vi "DevScripts_FlagToRing-Keycode.vi"() -> ()   [LabVIEW 2024]
uses:
  <vilib>/regexp/Match Regular Expression.xnode
panel:
  in  "flags (0)":u32(ring) items=["SDLK_UNKNOWN"=0, "SDLK_RETURN"=13, "SDLK_ESCAPE"=27, "SDLK_BACKSPACE"=8, "SDLK_TAB"=9, "SDLK_SPACE"=32, "SDLK_EXCLAIM"=33, "SDLK_DBLAPOSTROPHE"=34, "SDLK_HASH"=35, "SDLK_DOLLAR"=36, "SDLK_PERCENT"=37, "SDLK_AMPERSAND"=38, "SDLK_APOSTROPHE"=39, "SDLK_LEFTPAREN"=40, "SDLK_RIGHTPAREN"=41, "SDLK_ASTERISK"=42, "SDLK_PLUS"=43, "SDLK_COMMA"=44, "SDLK_MINUS"=45, "SDLK_PERIOD"=46, "SDLK_SLASH"=47, "SDLK_0"=48, "SDLK_1"=49, "SDLK_2"=50, "SDLK_3"=51, "SDLK_4"=52, "SDLK_5"=53, "SDLK_6"=54, "SDLK_7"=55, "SDLK_8"=56, "SDLK_9"=57, "SDLK_COLON"=58, "SDLK_SEMICOLON"=59, "SDLK_LESS"=60, "SDLK_EQUALS"=61, "SDLK_GREATER"=62, "SDLK_QUESTION"=63, "SDLK_AT"=64, "SDLK_LEFTBRACKET"=91, "SDLK_BACKSLASH"=92, "SDLK_RIGHTBRACKET"=93, "SDLK_CARET"=94, "SDLK_UNDERSCORE"=95, "SDLK_GRAVE"=96, "SDLK_A"=97, "SDLK_B"=98, "SDLK_C"=99, "SDLK_D"=100, "SDLK_E"=101, "SDLK_F"=102, "SDLK_G"=103, "SDLK_H"=104, "SDLK_I"=105, "SDLK_J"=106, "SDLK_K"=107, "SDLK_L"=108, "SDLK_M"=109, "SDLK_N"=110, "SDLK_O"=111, "SDLK_P"=112, "SDLK_Q"=113, "SDLK_R"=114, "SDLK_S"=115, "SDLK_T"=116, "SDLK_U"=117, "SDLK_V"=118, "SDLK_W"=119, "SDLK_X"=120, "SDLK_Y"=121, "SDLK_Z"=122, "SDLK_LEFTBRACE"=123, "SDLK_PIPE"=124, "SDLK_RIGHTBRACE"=125, "SDLK_TILDE"=126, "SDLK_DELETE"=127, "SDLK_PLUSMINUS"=177, "SDLK_CAPSLOCK"=1073741881, "SDLK_F1"=1073741882, "SDLK_F2"=1073741883, "SDLK_F3"=1073741884, "SDLK_F4"=1073741885, "SDLK_F5"=1073741886, "SDLK_F6"=1073741887, "SDLK_F7"=1073741888, "SDLK_F8"=1073741889, "SDLK_F9"=1073741890, "SDLK_F10"=1073741891, "SDLK_F11"=1073741892, "SDLK_F12"=1073741893, "SDLK_PRINTSCREEN"=1073741894, "SDLK_SCROLLLOCK"=1073741895, "SDLK_PAUSE"=1073741896, "SDLK_INSERT"=1073741897, "SDLK_HOME"=1073741898, "SDLK_PAGEUP"=1073741899, "SDLK_END"=1073741901, "SDLK_PAGEDOWN"=1073741902, "SDLK_RIGHT"=1073741903, "SDLK_LEFT"=1073741904, "SDLK_DOWN"=1073741905, "SDLK_UP"=1073741906, "SDLK_NUMLOCKCLEAR"=1073741907, "SDLK_KP_DIVIDE"=1073741908, "SDLK_KP_MULTIPLY"=1073741909, "SDLK_KP_MINUS"=1073741910, "SDLK_KP_PLUS"=1073741911, "SDLK_KP_ENTER"=1073741912, "SDLK_KP_1"=1073741913, "SDLK_KP_2"=1073741914, "SDLK_KP_3"=1073741915, "SDLK_KP_4"=1073741916, "SDLK_KP_5"=1073741917, "SDLK_KP_6"=1073741918, "SDLK_KP_7"=1073741919, "SDLK_KP_8"=1073741920, "SDLK_KP_9"=1073741921, "SDLK_KP_0"=1073741922, "SDLK_KP_PERIOD"=1073741923, "SDLK_APPLICATION"=1073741925, "SDLK_POWER"=1073741926, "SDLK_KP_EQUALS"=1073741927, "SDLK_F13"=1073741928, "SDLK_F14"=1073741929, "SDLK_F15"=1073741930, "SDLK_F16"=1073741931, "SDLK_F17"=1073741932, "SDLK_F18"=1073741933, "SDLK_F19"=1073741934, "SDLK_F20"=1073741935, "SDLK_F21"=1073741936, "SDLK_F22"=1073741937, "SDLK_F23"=1073741938, "SDLK_F24"=1073741939, "SDLK_EXECUTE"=1073741940, "SDLK_HELP"=1073741941, "SDLK_MENU"=1073741942, "SDLK_SELECT"=1073741943, "SDLK_STOP"=1073741944, "SDLK_AGAIN"=1073741945, "SDLK_UNDO"=1073741946, "SDLK_CUT"=1073741947, "SDLK_COPY"=1073741948, "SDLK_PASTE"=1073741949, "SDLK_FIND"=1073741950, "SDLK_MUTE"=1073741951, "SDLK_VOLUMEUP"=1073741952, "SDLK_VOLUMEDOWN"=1073741953, "SDLK_KP_COMMA"=1073741957, "SDLK_KP_EQUALSAS400"=1073741958, "SDLK_ALTERASE"=1073741977, "SDLK_SYSREQ"=1073741978, "SDLK_CANCEL"=1073741979, "SDLK_CLEAR"=1073741980, "SDLK_PRIOR"=1073741981, "SDLK_RETURN2"=1073741982, "SDLK_SEPARATOR"=1073741983, "SDLK_OUT"=1073741984, "SDLK_OPER"=1073741985, "SDLK_CLEARAGAIN"=1073741986, "SDLK_CRSEL"=1073741987, "SDLK_EXSEL"=1073741988, "SDLK_KP_00"=1073742000, "SDLK_KP_000"=1073742001, "SDLK_THOUSANDSSEPARATOR"=1073742002, "SDLK_DECIMALSEPARATOR"=1073742003, "SDLK_CURRENCYUNIT"=1073742004, "SDLK_CURRENCYSUBUNIT"=1073742005, "SDLK_KP_LEFTPAREN"=1073742006, "SDLK_KP_RIGHTPAREN"=1073742007, "SDLK_KP_LEFTBRACE"=1073742008, "SDLK_KP_RIGHTBRACE"=1073742009, "SDLK_KP_TAB"=1073742010, "SDLK_KP_BACKSPACE"=1073742011, "SDLK_KP_A"=1073742012, "SDLK_KP_B"=1073742013, "SDLK_KP_C"=1073742014, "SDLK_KP_D"=1073742015, "SDLK_KP_E"=1073742016, "SDLK_KP_F"=1073742017, "SDLK_KP_XOR"=1073742018, "SDLK_KP_POWER"=1073742019, "SDLK_KP_PERCENT"=1073742020, "SDLK_KP_LESS"=1073742021, "SDLK_KP_GREATER"=1073742022, "SDLK_KP_AMPERSAND"=1073742023, "SDLK_KP_DBLAMPERSAND"=1073742024, "SDLK_KP_VERTICALBAR"=1073742025, "SDLK_KP_DBLVERTICALBAR"=1073742026, "SDLK_KP_COLON"=1073742027, "SDLK_KP_HASH"=1073742028, "SDLK_KP_SPACE"=1073742029, "SDLK_KP_AT"=1073742030, "SDLK_KP_EXCLAM"=1073742031, "SDLK_KP_MEMSTORE"=1073742032, "SDLK_KP_MEMRECALL"=1073742033, "SDLK_KP_MEMCLEAR"=1073742034, "SDLK_KP_MEMADD"=1073742035, "SDLK_KP_MEMSUBTRACT"=1073742036, "SDLK_KP_MEMMULTIPLY"=1073742037, "SDLK_KP_MEMDIVIDE"=1073742038, "SDLK_KP_PLUSMINUS"=1073742039, "SDLK_KP_CLEAR"=1073742040, "SDLK_KP_CLEARENTRY"=1073742041, "SDLK_KP_BINARY"=1073742042, "SDLK_KP_OCTAL"=1073742043, "SDLK_KP_DECIMAL"=1073742044, "SDLK_KP_HEXADECIMAL"=1073742045, "SDLK_LCTRL"=1073742048, "SDLK_LSHIFT"=1073742049, "SDLK_LALT"=1073742050, "SDLK_LGUI"=1073742051, "SDLK_RCTRL"=1073742052, "SDLK_RSHIFT"=1073742053, "SDLK_RALT"=1073742054, "SDLK_RGUI"=1073742055, "SDLK_MODE"=1073742081, "SDLK_SLEEP"=1073742082, "SDLK_WAKE"=1073742083, "SDLK_CHANNEL_INCREMENT"=1073742084, "SDLK_CHANNEL_DECREMENT"=1073742085, "SDLK_MEDIA_PLAY"=1073742086, "SDLK_MEDIA_PAUSE"=1073742087, "SDLK_MEDIA_RECORD"=1073742088, "SDLK_MEDIA_FAST_FORWARD"=1073742089, "SDLK_MEDIA_REWIND"=1073742090, "SDLK_MEDIA_NEXT_TRACK"=1073742091, "SDLK_MEDIA_PREVIOUS_TRACK"=1073742092, "SDLK_MEDIA_STOP"=1073742093, "SDLK_MEDIA_EJECT"=1073742094, "SDLK_MEDIA_PLAY_PAUSE"=1073742095, "SDLK_MEDIA_SELECT"=1073742096, "SDLK_AC_NEW"=1073742097, "SDLK_AC_OPEN"=1073742098, "SDLK_AC_CLOSE"=1073742099, "SDLK_AC_EXIT"=1073742100, "SDLK_AC_SAVE"=1073742101, "SDLK_AC_PRINT"=1073742102, "SDLK_AC_PROPERTIES"=1073742103, "SDLK_AC_SEARCH"=1073742104, "SDLK_AC_HOME"=1073742105, "SDLK_AC_BACK"=1073742106, "SDLK_AC_FORWARD"=1073742107, "SDLK_AC_STOP"=1073742108, "SDLK_AC_REFRESH"=1073742109, "SDLK_AC_BOOKMARKS"=1073742110, "SDLK_SOFTLEFT"=1073742111, "SDLK_SOFTRIGHT"=1073742112, "SDLK_CALL"=1073742113, "SDLK_ENDCALL"=1073742114]
  in  "#Define list":string="#define SDLK_SCANCODE_MASK          (1u<<30)\n#define SDL_SCANCODE_TO_KEYCODE(X)  (X | SDLK_SCANCODE_MASK)\n#define SDLK_UNKNOWN                0x00000000u /**< 0 */\n#define SDLK_RETURN                 0x0000000du /**< '\\r' */\n#define SDLK_ESCAPE                 0x0000001bu /**< '\\x1B' */\n#define SDLK_BACKSPACE              0x00000008u /**< '\\b' */\n#define SDLK_TAB                    0x00000009u /**< '\\t' */\n#define SDLK_SPACE                  0x00000020u /**< ' ' */\n#define SDLK_EXCLAIM                0x00000021u /**< '!' */\n#define SDLK_DBLAPOSTROPHE          0x00000022u /**< '\"' */\n#define SDLK_HASH                   0x00000023u /**< '#' */\n#define SDLK_DOLLAR                 0x00000024u /**< '$' */\n#define SDLK_PERCENT                0x00000025u /**< '%' */\n#define SDLK_AMPERSAND              0x00000026u /**< '&' */\n#define SDLK_APOSTROPHE             0x00000027u /**< '\\'' */\n#define SDLK_LEFTPAREN              0x00000028u /**< '(' */\n#define SDLK_RIGHTPAREN             0x00000029u /**< ')' */\n#define SDLK_ASTERISK               0x0000002au /**< '*' */\n#define SDLK_PLUS                   0x0000002bu /**< '+' */\n#define SDLK_COMMA                  0x0000002cu /**< ',' */\n#define SDLK_MINUS                  0x0000002du /**< '-' */\n#define SDLK_PERIOD                 0x0000002eu /**< '.' */\n#define SDLK_SLASH                  0x0000002fu /**< '/' */\n#define SDLK_0                      0x00000030u /**< '0' */\n#define SDLK_1                      0x00000031u /**< '1' */\n#define SDLK_2                      0x00000032u /**< '2' */\n#define SDLK_3                      0x00000033u /**< '3' */\n#define SDLK_4                      0x00000034u /**< '4' */\n#define SDLK_5                      0x00000035u /**< '5' */\n#define SDLK_6                      0x00000036u /**< '6' */\n#define SDLK_7                      0x00000037u /**< '7' */\n#define SDLK_8                      0x00000038u /**< '8' */\n#define SDLK_9                      0x00000039u /**< '9' */\n#define SDLK_COLON                  0x0000003au /**< ':' */\n#define SDLK_SEMICOLON              0x0000003bu /**< ';' */\n#define SDLK_LESS                   0x0000003cu /**< '<' */\n#define SDLK_EQUALS                 0x0000003du /**< '=' */\n#define SDLK_GREATER                0x0000003eu /**< '>' */\n#define SDLK_QUESTION               0x0000003fu /**< '?' */\n#define SDLK_AT                     0x00000040u /**< '@' */\n#define SDLK_LEFTBRACKET            0x0000005bu /**< '[' */\n#define SDLK_BACKSLASH              0x0000005cu /**< '\\\\' */\n#define SDLK_RIGHTBRACKET           0x0000005du /**< ']' */\n#define SDLK_CARET                  0x0000005eu /**< '^' */\n#define SDLK_UNDERSCORE             0x0000005fu /**< '_' */\n#define SDLK_GRAVE                  0x00000060u /**< '`' */\n#define SDLK_A                      0x00000061u /**< 'a' */\n#define SDLK_B                      0x00000062u /**< 'b' */\n#define SDLK_C                      0x00000063u /**< 'c' */\n#define SDLK_D                      0x00000064u /**< 'd' */\n#define SDLK_E                      0x00000065u /**< 'e' */\n#define SDLK_F                      0x00000066u /**< 'f' */\n#define SDLK_G                      0x00000067u /**< 'g' */\n#define SDLK_H                      0x00000068u /**< 'h' */\n#define SDLK_I                      0x00000069u /**< 'i' */\n#define SDLK_J                      0x0000006au /**< 'j' */\n#define SDLK_K                      0x0000006bu /**< 'k' */\n#define SDLK_L                      0x0000006cu /**< 'l' */\n#define SDLK_M                      0x0000006du /**< 'm' */\n#define SDLK_N                      0x0000006eu /**< 'n' */\n#define SDLK_O                      0x0000006fu /**< 'o' */\n#define SDLK_P                      0x00000070u /**< 'p' */\n#define SDLK_Q                      0x00000071u /**< 'q' */\n#define SDLK_R                      0x00000072u /**< 'r' */\n#define SDLK_S                      0x00000073u /**< 's' */\n#define SDLK_T                      0x00000074u /**< 't' */\n#define SDLK_U                      0x00000075u /**< 'u' */\n#define SDLK_V                      0x00000076u /**< 'v' */\n#define SDLK_W                      0x00000077u /**< 'w' */\n#define SDLK_X                      0x00000078u /**< 'x' */\n#define SDLK_Y                      0x00000079u /**< 'y' */\n#define SDLK_Z                      0x0000007au /**< 'z' */\n#define SDLK_LEFTBRACE              0x0000007bu /**< '{' */\n#define SDLK_PIPE                   0x0000007cu /**< '|' */\n#define SDLK_RIGHTBRACE             0x0000007du /**< '}' */\n#define SDLK_TILDE                  0x0000007eu /**< '~' */\n#define SDLK_DELETE                 0x0000007fu /**< '\\x7F' */\n#define SDLK_PLUSMINUS              0x000000b1u /**< '\\xB1' */\n#define SDLK_CAPSLOCK               0x40000039u /**< SDL_SCANCODE_TO_KEYCODE(SDL_SCANCODE_CAPSLOCK) */\n#define SDLK_F1                     0x4000003au /**< SDL_SCANCODE_TO_KEYCODE(SDL_SCANCODE_F1) */\n#define SDLK_F2                     0x4000003bu /**< SDL_SCANCODE_TO_KEYCODE(SDL_SCANCODE_F2) */\n#define SDLK_F3                     0x4000003cu /**< SDL_SCANCODE_TO_KEYCODE(SDL_SCANCODE_F3) */\n#define SDLK_F4                     0x4000003du /**< SDL_SCANCODE_TO_KEYCODE(SDL_SCANCODE_F4) */\n#define SDLK_F5                     0x4000003eu /**< SDL_SCANCODE_TO_KEYCODE(SDL_SCANCODE_F5) */\n#define SDLK_F6                     0x4000003fu /**< SDL_SCANCODE_TO_KEYCODE(SDL_SCANCODE_F6) */\n#define SDLK_F7                     0x40000040u /**< SDL_SCANCODE_TO_KEYCODE(SDL_SCANCODE_F7) */\n#define SDLK_F8                     0x40000041u /**< SDL_SCANCODE_TO_KEYCODE(SDL_SCANCODE_F8) */\n#define SDLK_F9                     0x40000042u /**< SDL_SCANCODE_TO_KEYCODE(SDL_SCANCODE_F9) */\n#define SDLK_F10                    0x40000043u /**< SDL_SCANCODE_TO_KEYCODE(SDL_SCANCODE_F10) */\n#define SDLK_F11                    0x40000044u /**< SDL_SCANCODE_TO_KEYCODE(SDL_SCANCODE_F11) */\n#define SDLK_F12                    0x40000045u /**< SDL_SCANCODE_TO_KEYCODE(SDL_SCANCODE_F12) */\n#define SDLK_PRINTSCREEN            0x40000046u /**< SDL_SCANCODE_TO_KEYCODE(SDL_SCANCODE_PRINTSCREEN) */\n#define SDLK_SCROLLLOCK             0x40000047u /**< SDL_SCANCODE_TO_KEYCODE(SDL_SCANCODE_SCROLLLOCK) */\n#define SDLK_PAUSE                  0x40000048u /**< SDL_SCANCODE_TO_KEYCODE(SDL_SCANCODE_PAUSE) */\n#define SDLK_INSERT                 0x40000049u /**< SDL_SCANCODE_TO_KEYCODE(SDL_SCANCODE_INSERT) */\n#define SDLK_HOME                   0x4000004au /**< SDL_SCANCODE_TO_KEYCODE(SDL_SCANCODE_HOME) */\n#define SDLK_PAGEUP                 0x4000004bu /**< SDL_SCANCODE_TO_KEYCODE(SDL_SCANCODE_PAGEUP) */\n#define SDLK_END                    0x4000004du /**< SDL_SCANCODE_TO_KEYCODE(SDL_SCANCODE_END) */\n#define SDLK_PAGEDOWN               0x4000004eu /**< SDL_SCANCODE_TO_KEYCODE(SDL_SCANCODE_PAGEDOWN) */\n#define SDLK_RIGHT                  0x4000004fu /**< SDL_SCANCODE_TO_KEYCODE(SDL_SCANCODE_RIGHT) */\n#define SDLK_LEFT                   0x40000050u /**< SDL_SCANCODE_TO_KEYCODE(SDL_SCANCODE_LEFT) */\n#define SDLK_DOWN                   0x40000051u /**< SDL_SCANCODE_TO_KEYCODE(SDL_SCANCODE_DOWN) */\n#define SDLK_UP                     0x40000052u /**< SDL_SCANCODE_TO_KEYCODE(SDL_SCANCODE_UP) */\n#define SDLK_NUMLOCKCLEAR           0x40000053u /**< SDL_SCANCODE_TO_KEYCODE(SDL_SCANCODE_NUMLOCKCLEAR) */\n#define SDLK_KP_DIVIDE              0x40000054u /**< SDL_SCANCODE_TO_KEYCODE(SDL_SCANCODE_KP_DIVIDE) */\n#define SDLK_KP_MULTIPLY            0x40000055u /**< SDL_SCANCODE_TO_KEYCODE(SDL_SCANCODE_KP_MULTIPLY) */\n#define SDLK_KP_MINUS               0x40000056u /**< SDL_SCANCODE_TO_KEYCODE(SDL_SCANCODE_KP_MINUS) */\n#define SDLK_KP_PLUS                0x40000057u /**< SDL_SCANCODE_TO_KEYCODE(SDL_SCANCODE_KP_PLUS) */\n#define SDLK_KP_ENTER               0x40000058u /**< SDL_SCANCODE_TO_KEYCODE(SDL_SCANCODE_KP_ENTER) */\n#define SDLK_KP_1                   0x40000059u /**< SDL_SCANCODE_TO_KEYCODE(SDL_SCANCODE_KP_1) */\n#define SDLK_KP_2                   0x4000005au /**< SDL_SCANCODE_TO_KEYCODE(SDL_SCANCODE_KP_2) */\n#define SDLK_KP_3                   0x4000005bu /**< SDL_SCANCODE_TO_KEYCODE(SDL_SCANCODE_KP_3) */\n#define SDLK_KP_4                   0x4000005cu /**< SDL_SCANCODE_TO_KEYCODE(SDL_SCANCODE_KP_4) */\n#define SDLK_KP_5                   0x4000005du /**< SDL_SCANCODE_TO_KEYCODE(SDL_SCANCODE_KP_5) */\n#define SDLK_KP_6                   0x4000005eu /**< SDL_SCANCODE_TO_KEYCODE(SDL_SCANCODE_KP_6) */\n#define SDLK_KP_7                   0x4000005fu /**< SDL_SCANCODE_TO_KEYCODE(SDL_SCANCODE_KP_7) */\n#define SDLK_KP_8                   0x40000060u /**< SDL_SCANCODE_TO_KEYCODE(SDL_SCANCODE_KP_8) */\n#define SDLK_KP_9                   0x40000061u /**< SDL_SCANCODE_TO_KEYCODE(SDL_SCANCODE_KP_9) */\n#define SDLK_KP_0                   0x40000062u /**< SDL_SCANCODE_TO_KEYCODE(SDL_SCANCODE_KP_0) */\n#define SDLK_KP_PERIOD              0x40000063u /**< SDL_SCANCODE_TO_KEYCODE(SDL_SCANCODE_KP_PERIOD) */\n#define SDLK_APPLICATION            0x40000065u /**< SDL_SCANCODE_TO_KEYCODE(SDL_SCANCODE_APPLICATION) */\n#define SDLK_POWER                  0x40000066u /**< SDL_SCANCODE_TO_KEYCODE(SDL_SCANCODE_POWER) */\n#define SDLK_KP_EQUALS              0x40000067u /**< SDL_SCANCODE_TO_KEYCODE(SDL_SCANCODE_KP_EQUALS) */\n#define SDLK_F13                    0x40000068u /**< SDL_SCANCODE_TO_KEYCODE(SDL_SCANCODE_F13) */\n#define SDLK_F14                    0x40000069u /**< SDL_SCANCODE_TO_KEYCODE(SDL_SCANCODE_F14) */\n#define SDLK_F15                    0x4000006au /**< SDL_SCANCODE_TO_KEYCODE(SDL_SCANCODE_F15) */\n#define SDLK_F16                    0x4000006bu /**< SDL_SCANCODE_TO_KEYCODE(SDL_SCANCODE_F16) */\n#define SDLK_F17                    0x4000006cu /**< SDL_SCANCODE_TO_KEYCODE(SDL_SCANCODE_F17) */\n#define SDLK_F18                    0x4000006du /**< SDL_SCANCODE_TO_KEYCODE(SDL_SCANCODE_F18) */\n#define SDLK_F19                    0x4000006eu /**< SDL_SCANCODE_TO_KEYCODE(SDL_SCANCODE_F19) */\n#define SDLK_F20                    0x4000006fu /**< SDL_SCANCODE_TO_KEYCODE(SDL_SCANCODE_F20) */\n#define SDLK_F21                    0x40000070u /**< SDL_SCANCODE_TO_KEYCODE(SDL_SCANCODE_F21) */\n#define SDLK_F22                    0x40000071u /**< SDL_SCANCODE_TO_KEYCODE(SDL_SCANCODE_F22) */\n#define SDLK_F23                    0x40000072u /**< SDL_SCANCODE_TO_KEYCODE(SDL_SCANCODE_F23) */\n#define SDLK_F24                    0x40000073u /**< SDL_SCANCODE_TO_KEYCODE(SDL_SCANCODE_F24) */\n#define SDLK_EXECUTE                0x40000074u /**< SDL_SCANCODE_TO_KEYCODE(SDL_SCANCODE_EXECUTE) */\n#define SDLK_HELP                   0x40000075u /**< SDL_SCANCODE_TO_KEYCODE(SDL_SCANCODE_HELP) */\n#define SDLK_MENU                   0x40000076u /**< SDL_SCANCODE_TO_KEYCODE(SDL_SCANCODE_MENU) */\n#define SDLK_SELECT                 0x40000077u /**< SDL_SCANCODE_TO_KEYCODE(SDL_SCANCODE_SELECT) */\n#define SDLK_STOP                   0x40000078u /**< SDL_SCANCODE_TO_KEYCODE(SDL_SCANCODE_STOP) */\n#define SDLK_AGAIN                  0x40000079u /**< SDL_SCANCODE_TO_KEYCODE(SDL_SCANCODE_AGAIN) */\n#define SDLK_UNDO                   0x4000007au /**< SDL_SCANCODE_TO_KEYCODE(SDL_SCANCODE_UNDO) */\n#define SDLK_CUT                    0x4000007bu /**< SDL_SCANCODE_TO_KEYCODE(SDL_SCANCODE_CUT) */\n#define SDLK_COPY                   0x4000007cu /**< SDL_SCANCODE_TO_KEYCODE(SDL_SCANCODE_COPY) */\n#define SDLK_PASTE                  0x4000007du /**< SDL_SCANCODE_TO_KEYCODE(SDL_SCANCODE_PASTE) */\n#define SDLK_FIND                   0x4000007eu /**< SDL_SCANCODE_TO_KEYCODE(SDL_SCANCODE_FIND) */\n#define SDLK_MUTE                   0x4000007fu /**< SDL_SCANCODE_TO_KEYCODE(SDL_SCANCODE_MUTE) */\n#define SDLK_VOLUMEUP               0x40000080u /**< SDL_SCANCODE_TO_KEYCODE(SDL_SCANCODE_VOLUMEUP) */\n#define SDLK_VOLUMEDOWN             0x40000081u /**< SDL_SCANCODE_TO_KEYCODE(SDL_SCANCODE_VOLUMEDOWN) */\n#define SDLK_KP_COMMA               0x40000085u /**< SDL_SCANCODE_TO_KEYCODE(SDL_SCANCODE_KP_COMMA) */\n#define SDLK_KP_EQUALSAS400         0x40000086u /**< SDL_SCANCODE_TO_KEYCODE(SDL_SCANCODE_KP_EQUALSAS400) */\n#define SDLK_ALTERASE               0x40000099u /**< SDL_SCANCODE_TO_KEYCODE(SDL_SCANCODE_ALTERASE) */\n#define SDLK_SYSREQ                 0x4000009au /**< SDL_SCANCODE_TO_KEYCODE(SDL_SCANCODE_SYSREQ) */\n#define SDLK_CANCEL                 0x4000009bu /**< SDL_SCANCODE_TO_KEYCODE(SDL_SCANCODE_CANCEL) */\n#define SDLK_CLEAR                  0x4000009cu /**< SDL_SCANCODE_TO_KEYCODE(SDL_SCANCODE_CLEAR) */\n#define SDLK_PRIOR                  0x4000009du /**< SDL_SCANCODE_TO_KEYCODE(SDL_SCANCODE_PRIOR) */\n#define SDLK_RETURN2                0x4000009eu /**< SDL_SCANCODE_TO_KEYCODE(SDL_SCANCODE_RETURN2) */\n#define SDLK_SEPARATOR              0x4000009fu /**< SDL_SCANCODE_TO_KEYCODE(SDL_SCANCODE_SEPARATOR) */\n#define SDLK_OUT                    0x400000a0u /**< SDL_SCANCODE_TO_KEYCODE(SDL_SCANCODE_OUT) */\n#define SDLK_OPER                   0x400000a1u /**< SDL_SCANCODE_TO_KEYCODE(SDL_SCANCODE_OPER) */\n#define SDLK_CLEARAGAIN             0x400000a2u /**< SDL_SCANCODE_TO_KEYCODE(SDL_SCANCODE_CLEARAGAIN) */\n#define SDLK_CRSEL                  0x400000a3u /**< SDL_SCANCODE_TO_KEYCODE(SDL_SCANCODE_CRSEL) */\n#define SDLK_EXSEL                  0x400000a4u /**< SDL_SCANCODE_TO_KEYCODE(SDL_SCANCODE_EXSEL) */\n#define SDLK_KP_00                  0x400000b0u /**< SDL_SCANCODE_TO_KEYCODE(SDL_SCANCODE_KP_00) */\n#define SDLK_KP_000                 0x400000b1u /**< SDL_SCANCODE_TO_KEYCODE(SDL_SCANCODE_KP_000) */\n#define SDLK_THOUSANDSSEPARATOR     0x400000b2u /**< SDL_SCANCODE_TO_KEYCODE(SDL_SCANCODE_THOUSANDSSEPARATOR) */\n#define SDLK_DECIMALSEPARATOR       0x400000b3u /**< SDL_SCANCODE_TO_KEYCODE(SDL_SCANCODE_DECIMALSEPARATOR) */\n#define SDLK_CURRENCYUNIT           0x400000b4u /**< SDL_SCANCODE_TO_KEYCODE(SDL_SCANCODE_CURRENCYUNIT) */\n#define SDLK_CURRENCYSUBUNIT        0x400000b5u /**< SDL_SCANCODE_TO_KEYCODE(SDL_SCANCODE_CURRENCYSUBUNIT) */\n#define SDLK_KP_LEFTPAREN           0x400000b6u /**< SDL_SCANCODE_TO_KEYCODE(SDL_SCANCODE_KP_LEFTPAREN) */\n#define SDLK_KP_RIGHTPAREN          0x400000b7u /**< SDL_SCANCODE_TO_KEYCODE(SDL_SCANCODE_KP_RIGHTPAREN) */\n#define SDLK_KP_LEFTBRACE           0x400000b8u /**< SDL_SCANCODE_TO_KEYCODE(SDL_SCANCODE_KP_LEFTBRACE) */\n#define SDLK_KP_RIGHTBRACE          0x400000b9u /**< SDL_SCANCODE_TO_KEYCODE(SDL_SCANCODE_KP_RIGHTBRACE) */\n#define SDLK_KP_TAB                 0x400000bau /**< SDL_SCANCODE_TO_KEYCODE(SDL_SCANCODE_KP_TAB) */\n#define SDLK_KP_BACKSPACE           0x400000bbu /**< SDL_SCANCODE_TO_KEYCODE(SDL_SCANCODE_KP_BACKSPACE) */\n#define SDLK_KP_A                   0x400000bcu /**< SDL_SCANCODE_TO_KEYCODE(SDL_SCANCODE_KP_A) */\n#define SDLK_KP_B                   0x400000bdu /**< SDL_SCANCODE_TO_KEYCODE(SDL_SCANCODE_KP_B) */\n#define SDLK_KP_C                   0x400000beu /**< SDL_SCANCODE_TO_KEYCODE(SDL_SCANCODE_KP_C) */\n#define SDLK_KP_D                   0x400000bfu /**< SDL_SCANCODE_TO_KEYCODE(SDL_SCANCODE_KP_D) */\n#define SDLK_KP_E                   0x400000c0u /**< SDL_SCANCODE_TO_KEYCODE(SDL_SCANCODE_KP_E) */\n#define SDLK_KP_F                   0x400000c1u /**< SDL_SCANCODE_TO_KEYCODE(SDL_SCANCODE_KP_F) */\n#define SDLK_KP_XOR                 0x400000c2u /**< SDL_SCANCODE_TO_KEYCODE(SDL_SCANCODE_KP_XOR) */\n#define SDLK_KP_POWER               0x400000c3u /**< SDL_SCANCODE_TO_KEYCODE(SDL_SCANCODE_KP_POWER) */\n#define SDLK_KP_PERCENT             0x400000c4u /**< SDL_SCANCODE_TO_KEYCODE(SDL_SCANCODE_KP_PERCENT) */\n#define SDLK_KP_LESS                0x400000c5u /**< SDL_SCANCODE_TO_KEYCODE(SDL_SCANCODE_KP_LESS) */\n#define SDLK_KP_GREATER             0x400000c6u /**< SDL_SCANCODE_TO_KEYCODE(SDL_SCANCODE_KP_GREATER) */\n#define SDLK_KP_AMPERSAND           0x400000c7u /**< SDL_SCANCODE_TO_KEYCODE(SDL_SCANCODE_KP_AMPERSAND) */\n#define SDLK_KP_DBLAMPERSAND        0x400000c8u /**< SDL_SCANCODE_TO_KEYCODE(SDL_SCANCODE_KP_DBLAMPERSAND) */\n#define SDLK_KP_VERTICALBAR         0x400000c9u /**< SDL_SCANCODE_TO_KEYCODE(SDL_SCANCODE_KP_VERTICALBAR) */\n#define SDLK_KP_DBLVERTICALBAR      0x400000cau /**< SDL_SCANCODE_TO_KEYCODE(SDL_SCANCODE_KP_DBLVERTICALBAR) */\n#define SDLK_KP_COLON               0x400000cbu /**< SDL_SCANCODE_TO_KEYCODE(SDL_SCANCODE_KP_COLON) */\n#define SDLK_KP_HASH                0x400000ccu /**< SDL_SCANCODE_TO_KEYCODE(SDL_SCANCODE_KP_HASH) */\n#define SDLK_KP_SPACE               0x400000cdu /**< SDL_SCANCODE_TO_KEYCODE(SDL_SCANCODE_KP_SPACE) */\n#define SDLK_KP_AT                  0x400000ceu /**< SDL_SCANCODE_TO_KEYCODE(SDL_SCANCODE_KP_AT) */\n#define SDLK_KP_EXCLAM              0x400000cfu /**< SDL_SCANCODE_TO_KEYCODE(SDL_SCANCODE_KP_EXCLAM) */\n#define SDLK_KP_MEMSTORE            0x400000d0u /**< SDL_SCANCODE_TO_KEYCODE(SDL_SCANCODE_KP_MEMSTORE) */\n#define SDLK_KP_MEMRECALL           0x400000d1u /**< SDL_SCANCODE_TO_KEYCODE(SDL_SCANCODE_KP_MEMRECALL) */\n#define SDLK_KP_MEMCLEAR            0x400000d2u /**< SDL_SCANCODE_TO_KEYCODE(SDL_SCANCODE_KP_MEMCLEAR) */\n#define SDLK_KP_MEMADD              0x400000d3u /**< SDL_SCANCODE_TO_KEYCODE(SDL_SCANCODE_KP_MEMADD) */\n#define SDLK_KP_MEMSUBTRACT         0x400000d4u /**< SDL_SCANCODE_TO_KEYCODE(SDL_SCANCODE_KP_MEMSUBTRACT) */\n#define SDLK_KP_MEMMULTIPLY         0x400000d5u /**< SDL_SCANCODE_TO_KEYCODE(SDL_SCANCODE_KP_MEMMULTIPLY) */\n#define SDLK_KP_MEMDIVIDE           0x400000d6u /**< SDL_SCANCODE_TO_KEYCODE(SDL_SCANCODE_KP_MEMDIVIDE) */\n#define SDLK_KP_PLUSMINUS           0x400000d7u /**< SDL_SCANCODE_TO_KEYCODE(SDL_SCANCODE_KP_PLUSMINUS) */\n#define SDLK_KP_CLEAR               0x400000d8u /**< SDL_SCANCODE_TO_KEYCODE(SDL_SCANCODE_KP_CLEAR) */\n#define SDLK_KP_CLEARENTRY          0x400000d9u /**< SDL_SCANCODE_TO_KEYCODE(SDL_SCANCODE_KP_CLEARENTRY) */\n#define SDLK_KP_BINARY              0x400000dau /**< SDL_SCANCODE_TO_KEYCODE(SDL_SCANCODE_KP_BINARY) */\n#define SDLK_KP_OCTAL               0x400000dbu /**< SDL_SCANCODE_TO_KEYCODE(SDL_SCANCODE_KP_OCTAL) */\n#define SDLK_KP_DECIMAL             0x400000dcu /**< SDL_SCANCODE_TO_KEYCODE(SDL_SCANCODE_KP_DECIMAL) */\n#define SDLK_KP_HEXADECIMAL         0x400000ddu /**< SDL_SCANCODE_TO_KEYCODE(SDL_SCANCODE_KP_HEXADECIMAL) */\n#define SDLK_LCTRL                  0x400000e0u /**< SDL_SCANCODE_TO_KEYCODE(SDL_SCANCODE_LCTRL) */\n#define SDLK_LSHIFT                 0x400000e1u /**< SDL_SCANCODE_TO_KEYCODE(SDL_SCANCODE_LSHIFT) */\n#define SDLK_LALT                   0x400000e2u /**< SDL_SCANCODE_TO_KEYCODE(SDL_SCANCODE_LALT) */\n#define SDLK_LGUI                   0x400000e3u /**< SDL_SCANCODE_TO_KEYCODE(SDL_SCANCODE_LGUI) */\n#define SDLK_RCTRL                  0x400000e4u /**< SDL_SCANCODE_TO_KEYCODE(SDL_SCANCODE_RCTRL) */\n#define SDLK_RSHIFT                 0x400000e5u /**< SDL_SCANCODE_TO_KEYCODE(SDL_SCANCODE_RSHIFT) */\n#define SDLK_RALT                   0x400000e6u /**< SDL_SCANCODE_TO_KEYCODE(SDL_SCANCODE_RALT) */\n#define SDLK_RGUI                   0x400000e7u /**< SDL_SCANCODE_TO_KEYCODE(SDL_SCANCODE_RGUI) */\n#define SDLK_MODE                   0x40000101u /**< SDL_SCANCODE_TO_KEYCODE(SDL_SCANCODE_MODE) */\n#define SDLK_SLEEP                  0x40000102u /**< SDL_SCANCODE_TO_KEYCODE(SDL_SCANCODE_SLEEP) */\n#define SDLK_WAKE                   0x40000103u /**< SDL_SCANCODE_TO_KEYCODE(SDL_SCANCODE_WAKE) */\n#define SDLK_CHANNEL_INCREMENT      0x40000104u /**< SDL_SCANCODE_TO_KEYCODE(SDL_SCANCODE_CHANNEL_INCREMENT) */\n#define SDLK_CHANNEL_DECREMENT      0x40000105u /**< SDL_SCANCODE_TO_KEYCODE(SDL_SCANCODE_CHANNEL_DECREMENT) */\n#define SDLK_MEDIA_PLAY             0x40000106u /**< SDL_SCANCODE_TO_KEYCODE(SDL_SCANCODE_MEDIA_PLAY) */\n#define SDLK_MEDIA_PAUSE            0x40000107u /**< SDL_SCANCODE_TO_KEYCODE(SDL_SCANCODE_MEDIA_PAUSE) */\n#define SDLK_MEDIA_RECORD           0x40000108u /**< SDL_SCANCODE_TO_KEYCODE(SDL_SCANCODE_MEDIA_RECORD) */\n#define SDLK_MEDIA_FAST_FORWARD     0x40000109u /**< SDL_SCANCODE_TO_KEYCODE(SDL_SCANCODE_MEDIA_FAST_FORWARD) */\n#define SDLK_MEDIA_REWIND           0x4000010au /**< SDL_SCANCODE_TO_KEYCODE(SDL_SCANCODE_MEDIA_REWIND) */\n#define SDLK_MEDIA_NEXT_TRACK       0x4000010bu /**< SDL_SCANCODE_TO_KEYCODE(SDL_SCANCODE_MEDIA_NEXT_TRACK) */\n#define SDLK_MEDIA_PREVIOUS_TRACK   0x4000010cu /**< SDL_SCANCODE_TO_KEYCODE(SDL_SCANCODE_MEDIA_PREVIOUS_TRACK) */\n#define SDLK_MEDIA_STOP             0x4000010du /**< SDL_SCANCODE_TO_KEYCODE(SDL_SCANCODE_MEDIA_STOP) */\n#define SDLK_MEDIA_EJECT            0x4000010eu /**< SDL_SCANCODE_TO_KEYCODE(SDL_SCANCODE_MEDIA_EJECT) */\n#define SDLK_MEDIA_PLAY_PAUSE       0x4000010fu /**< SDL_SCANCODE_TO_KEYCODE(SDL_SCANCODE_MEDIA_PLAY_PAUSE) */\n#define SDLK_MEDIA_SELECT           0x40000110u /**< SDL_SCANCODE_TO_KEYCODE(SDL_SCANCODE_MEDIA_SELECT) */\n#define SDLK_AC_NEW                 0x40000111u /**< SDL_SCANCODE_TO_KEYCODE(SDL_SCANCODE_AC_NEW) */\n#define SDLK_AC_OPEN                0x40000112u /**< SDL_SCANCODE_TO_KEYCODE(SDL_SCANCODE_AC_OPEN) */\n#define SDLK_AC_CLOSE               0x40000113u /**< SDL_SCANCODE_TO_KEYCODE(SDL_SCANCODE_AC_CLOSE) */\n#define SDLK_AC_EXIT                0x40000114u /**< SDL_SCANCODE_TO_KEYCODE(SDL_SCANCODE_AC_EXIT) */\n#define SDLK_AC_SAVE                0x40000115u /**< SDL_SCANCODE_TO_KEYCODE(SDL_SCANCODE_AC_SAVE) */\n#define SDLK_AC_PRINT               0x40000116u /**< SDL_SCANCODE_TO_KEYCODE(SDL_SCANCODE_AC_PRINT) */\n#define SDLK_AC_PROPERTIES          0x40000117u /**< SDL_SCANCODE_TO_KEYCODE(SDL_SCANCODE_AC_PROPERTIES) */\n#define SDLK_AC_SEARCH              0x40000118u /**< SDL_SCANCODE_TO_KEYCODE(SDL_SCANCODE_AC_SEARCH) */\n#define SDLK_AC_HOME                0x40000119u /**< SDL_SCANCODE_TO_KEYCODE(SDL_SCANCODE_AC_HOME) */\n#define SDLK_AC_BACK                0x4000011au /**< SDL_SCANCODE_TO_KEYCODE(SDL_SCANCODE_AC_BACK) */\n#define SDLK_AC_FORWARD             0x4000011bu /**< SDL_SCANCODE_TO_KEYCODE(SDL_SCANCODE_AC_FORWARD) */\n#define SDLK_AC_STOP                0x4000011cu /**< SDL_SCANCODE_TO_KEYCODE(SDL_SCANCODE_AC_STOP) */\n#define SDLK_AC_REFRESH             0x4000011du /**< SDL_SCANCODE_TO_KEYCODE(SDL_SCANCODE_AC_REFRESH) */\n#define SDLK_AC_BOOKMARKS           0x4000011eu /**< SDL_SCANCODE_TO_KEYCODE(SDL_SCANCODE_AC_BOOKMARKS) */\n#define SDLK_SOFTLEFT               0x4000011fu /**< SDL_SCANCODE_TO_KEYCODE(SDL_SCANCODE_SOFTLEFT) */\n#define SDLK_SOFTRIGHT              0x40000120u /**< SDL_SCANCODE_TO_KEYCODE(SDL_SCANCODE_SOFTRIGHT) */\n#define SDLK_CALL                   0x40000121u /**< SDL_SCANCODE_TO_KEYCODE(SDL_SCANCODE_CALL) */\n#define SDLK_ENDCALL                0x40000122u /**< SDL_SCANCODE_TO_KEYCODE(SDL_SCANCODE_ENDCALL) */"
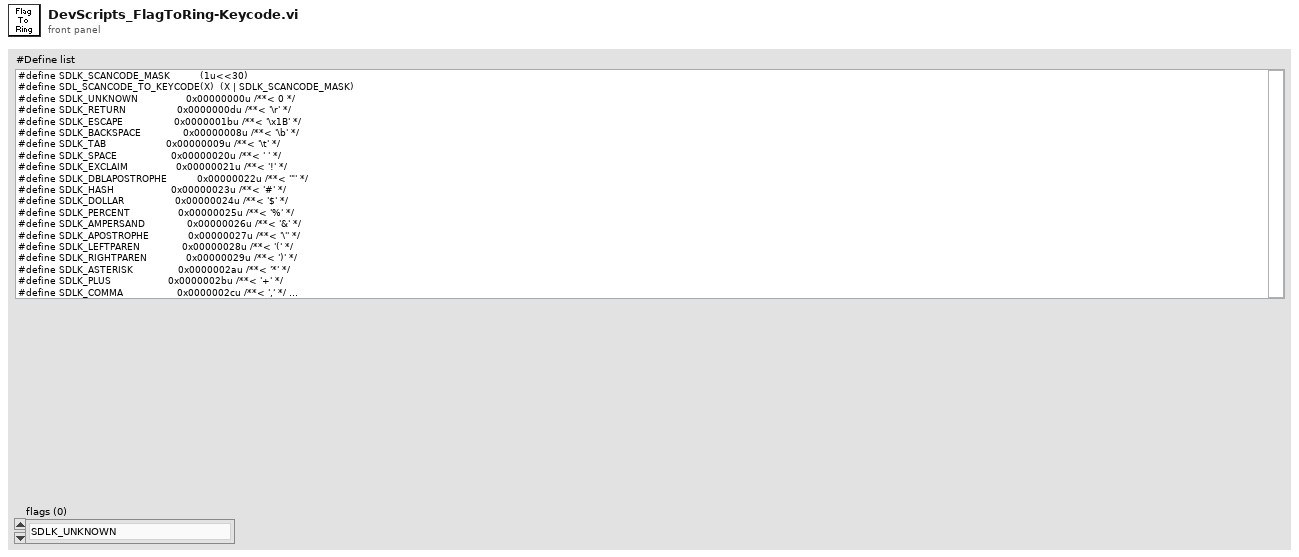
[diagram p1: front panel]
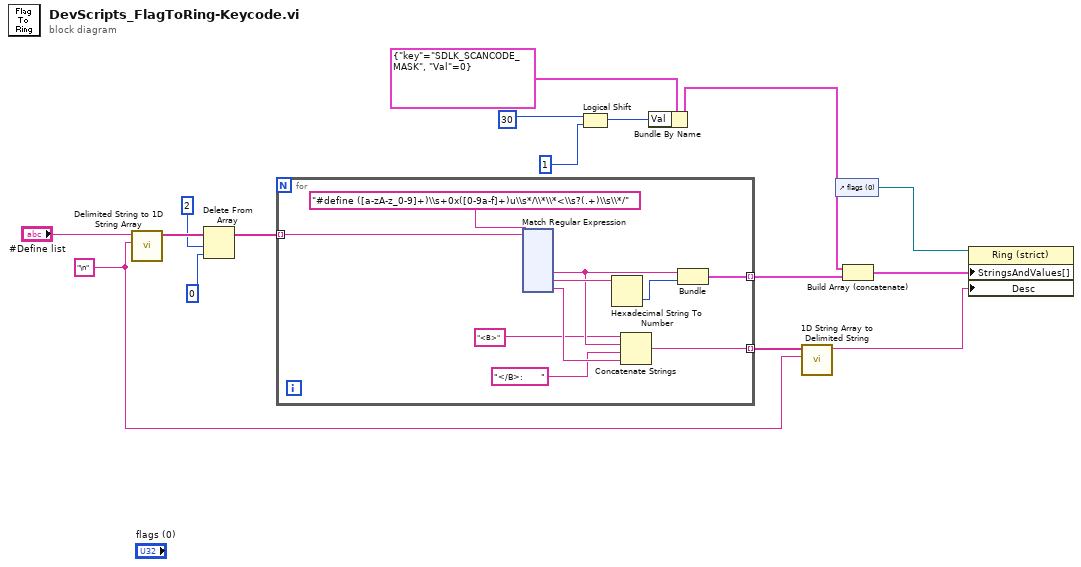
[diagram p0: block diagram]
diagram:
  w12 = "\n" ("delimiter")
  n1 = call <vilib>:"Delimited String to 1D String Array.vi"("delimiter"=w12, "delimited string"="#Define list") -> ("string array"=w15:string[])  [unwired: 9 in]
  n2 = Delete From Array(array=w15, length=2, index=0) -> (array with subset deleted=w8:string[])  [unwired: 1 out]
  n3 = for {
    tunnel: w8 -> [w26] mode=indexing
    tunnel: [w23] -> w14 mode=indexing
    tunnel: [w19] -> w13 mode=indexing
    n4 = xnode "Match Regular Expression"("input string"=w26, "regular expression"="#define ([a-zA-z_0-9]+)\\s+0x([0-9a-f]+)u\\s*/\\*\\*<\\s?(.+)\\s\\*/") -> ("submatch 1"=w21:string, "submatch 2"=w24:string, "submatch 3"=w20:string)  [unwired: 4 in, 5 out]
    n5 = Hexadecimal String To Number(string=w24) -> (number=w22:u32)  [unwired: 2 in, 1 out]
    n6 = Concatenate Strings("<B>" ("string"), w21, "</B>:      " ("string"), w20) -> (w19:string)
    n7 = Bundle("submatch 1"=w21, w22) -> (w23:cluster{"submatch 1":string, u32})  [unwired: 1 in]
  }
  n8 = Logical Shift(y=u32 30, x=u32 1) -> (x << y=w1:u32)
  n9 = Bundle By Name(cluster=cluster{"key":string, "Val":u32} {"key"="SDLK_SCANCODE_MASK", "Val"=0}, "Val"=w1) -> (w4:cluster{"key":string, "Val":u32})
  n10 = call <vilib>:"1D String Array to Delimited String.vi"("delimiter"=w12, "string array"=w13) -> ("delimited string"=w9:string)  [unwired: 9 in]
  n11 = control-ref of="flags (0)"() -> (w11:refnum<vi>)
  n12 = Build Array (concatenate)(w4, w14) -> (w10:cluster{"submatch 1":string, "Val":u32}[])
  n13 = property class="Ring (strict)"(reference=w11, "StringsAndValues[]"=w10, "Desc"=w9) -> ()  [unwired: 1 in, 2 out]
